vi "PPR_SIM_SIM_ODOM_FIELD_CLAMP.vi"(9 "in SWERVE_DRIVE_ODOMETRY":T1={"M_POSE_Meters"={"TRANSLATION"={"X"=0.0, "Y"=0.0}, "ROTATION"={"VALUE"=0.0, "COS"=1.0, "SIN"=0.0}}, "M_GyroOffset"={"VALUE"=0.0, "COS"=1.0, "SIN"=0.0}, "M_PrevAngle"={"VALUE"=0.0, "COS"=1.0, "SIN"=0.0}, "M_PrevLeftDist_M"=0.0, "M_PrevRightDist_M"=0.0, "M_InitLeftDist_M"=0.0, "M_InitRightDist_M"=0.0} {"M_PrevAngle"."SIN" format="%13.4f"; "M_PrevAngle"."COS" format="%13.4f"; "M_PrevAngle"."VALUE" format="%13.4f"; "M_GyroOffset"."SIN" format="%13.4f"; "M_GyroOffset"."COS" format="%13.4f"; "M_GyroOffset"."VALUE" format="%13.4f"; "M_POSE_Meters"."ROTATION"."SIN" format="%13.4f"; "M_POSE_Meters"."ROTATION"."COS" format="%13.4f"; "M_POSE_Meters"."ROTATION"."VALUE" format="%13.4f"; "M_POSE_Meters"."TRANSLATION"."Y" format="%14.3f"; "M_POSE_Meters"."TRANSLATION"."X" format="%14.3f"}) -> (1 "out SWERVE_DRIVE_ODOMETRY":T1={"M_POSE_Meters"={"TRANSLATION"={"X"=0.0, "Y"=0.0}, "ROTATION"={"VALUE"=0.0, "COS"=1.0, "SIN"=0.0}}, "M_GyroOffset"={"VALUE"=0.0, "COS"=1.0, "SIN"=0.0}, "M_PrevAngle"={"VALUE"=0.0, "COS"=1.0, "SIN"=0.0}, "M_PrevLeftDist_M"=0.0, "M_PrevRightDist_M"=0.0, "M_InitLeftDist_M"=0.0, "M_InitRightDist_M"=0.0} {"M_PrevAngle"."SIN" format="%13.4f"; "M_PrevAngle"."COS" format="%13.4f"; "M_PrevAngle"."VALUE" format="%13.4f"; "M_GyroOffset"."SIN" format="%13.4f"; "M_GyroOffset"."COS" format="%13.4f"; "M_GyroOffset"."VALUE" format="%13.4f"; "M_POSE_Meters"."ROTATION"."SIN" format="%13.4f"; "M_POSE_Meters"."ROTATION"."COS" format="%13.4f"; "M_POSE_Meters"."ROTATION"."VALUE" format="%13.4f"; "M_POSE_Meters"."TRANSLATION"."Y" format="%14.3f"; "M_POSE_Meters"."TRANSLATION"."X" format="%14.3f"})   [LabVIEW 2019]
uses:
  <vilib>/Rock Robotics/WPI/ThirdParty/JAS_Junk/TrajLib/TypeDef/DIFF_DRIVE_ODOM2.ctl
  <vilib>/Rock Robotics/WPI/ThirdParty/JAS_Junk/TrajLib/TypeDef/POSE2D.ctl
  <vilib>/Rock Robotics/WPI/ThirdParty/JAS_Junk/TrajLib/TypeDef/TRANSLATION2D.ctl
  <vilib>/Rock Robotics/WPI/ThirdParty/JAS_Junk/TrajLib/TypeDef/ROTATION2D.ctl
  <vilib>/Rock Robotics/WPI/ThirdParty/JAS_Junk/TrajLib/Trajectory_Library.lvlib
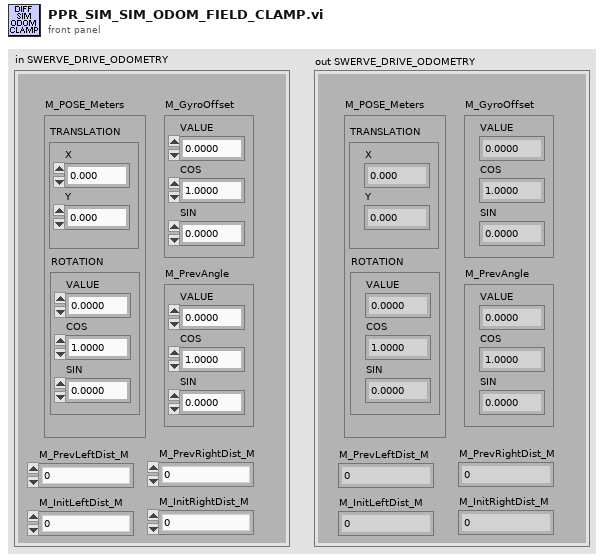
[diagram p1: front panel]
types:
  T1 = typedef "Trajectory_Library.lvlib/DIFF_DRIVE_ODOM2.ctl" = cluster{"M_POSE_Meters":T2, "M_GyroOffset":T4, "M_PrevAngle":T4, "M_PrevLeftDist_M":dbl, "M_PrevRightDist_M":dbl, "M_InitLeftDist_M":dbl, "M_InitRightDist_M":dbl}
  T2 = typedef "Trajectory_Library.lvlib/POSE2D.ctl" = cluster{"TRANSLATION":T3, "ROTATION":T4}
  T3 = typedef "Trajectory_Library.lvlib/TRANSLATION2D.ctl" = cluster{"X":dbl, "Y":dbl}
  T4 = typedef "Trajectory_Library.lvlib/ROTATION2D.ctl" = cluster{"VALUE":dbl, "COS":dbl, "SIN":dbl}
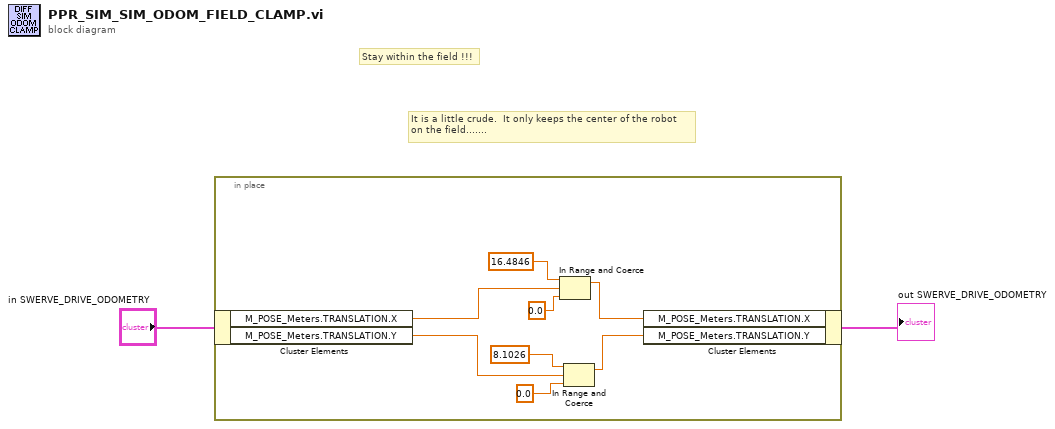
[diagram p0: block diagram]
diagram:
  # "It is a little crude.  It only keeps the center of the robot\non the field......."
  # "Stay within the field !!!"
  n1 = in-place {
    n2 = in-place-cluster #1("in SWERVE_DRIVE_ODOMETRY") -> ("M_POSE_Meters.TRANSLATION.X"=w8:dbl, "M_POSE_Meters.TRANSLATION.Y"=w9:dbl)
    n3 = In Range and Coerce(upper limit=16.4846, x=w8, lower limit=0.0) -> (coerced(x)=w10:dbl)  [unwired: 1 out]
    n4 = In Range and Coerce(upper limit=8.1026, x=w9, lower limit=0.0) -> (coerced(x)=w3:dbl)  [unwired: 1 out]
    n5 = in-place-cluster #1("M_POSE_Meters.TRANSLATION.X"=w10, "M_POSE_Meters.TRANSLATION.Y"=w3) -> (→"out SWERVE_DRIVE_ODOMETRY":T1)
  }
